vi "LJStreamM.vi"() -> ()   [LabVIEW 2025]
uses:
  LJstreamM globals.vi
panel:
  out "Meter 8":dbl(knob) scale=0.0..1000.0
  out "Meter 7":dbl(knob) scale=0.0..1000.0
  out "Meter 6":dbl(knob) scale=0.0..1000.0
  out "Meter 5":dbl(knob) scale=0.0..1000.0
  out "Meter 4":dbl(knob) scale=0.0..1000.0
  out "Meter 3":dbl(knob) scale=0.0..1000.0
  out "Meter 2":dbl(knob) scale=0.0..1000.0
  out "Meter":dbl(knob) scale=0.0..1000.0
  in  "Fire Button":bool
  in  "Open\nSolenoid":bool
  in  "Close Solenoid":bool
  in  "HIGH":dbl=1.0
  in  "Low":dbl
  in  "FIO6":string="FIO6"
  in  "Close\n Button":bool
  in  "PWM Output 1":string="DIO0_EF_CONFIG_A"
  in  "PWM Output 2":string="DIO2_EF_CONFIG_A"
  in  "Close":dbl=125000.0
  in  "Open":dbl=200000.0
  in  "Open Button":bool
  in  "Config Names":string[](array[string])=["AIN0_RANGE", "AIN0_RESOLUTION_INDEX", "DIO0_EF_ENABLE", "DIO_EF_CLOCK0_ENABLE", "DIO_EF_CLOCK0_ROLL_VALUE", "DIO0_EF_INDEX", "DIO_EF_CLOCK0_ENABLE", "DIO0_EF_ENABLE", "DIO2_EF_ENABLE", "DIO2_EF_INDEX", "DIO2_EF_ENABLE"]
  in  "Config Values":dbl[](array[numeric])=[10.0, 0.0, 0.0, 0.0, 800000.0, 0.0, 1.0, 1.0, 0.0, 0.0, 1.0] format="%.2f"
  out "SerialNumber":i32=470023915
  out "ConnType":i32=1
  out "DevType":i32=7
  in  "Select New Configs":bool
  in  "Save Configuration":bool
  out "Last Command-Response Error Message":string="No Error"
  in  "Change Working Directory":bool
  in  "Max File Size (Bytes)":i32=1048576 min=1 max=2000000000
  in  "Graph?":bool[](array[boolean])=[TRUE, TRUE, TRUE, TRUE, TRUE, TRUE, TRUE, TRUE, FALSE, FALSE, FALSE, FALSE, FALSE, FALSE, FALSE, FALSE]
  out "Scaled":dbl[](array[numeric])=[-2747.1556396198275, -2757.890681247711, -2748.909975194931, -2750.96038772583, -2759.144604291916, -2761.5666391944883, -2777.2834499549863, -2778.0301016235353, -10.5811185836792, -10.5811185836792, -10.581039428710938, -10.581039428710938, -10.581039428710938, -10.5811185836792] format="%.6f"
  in  "Scaling Equation":string[](array[string])=["y = 247.67*a - 126.53", "y = 248.78*b - 125.52", "y = 247.97*c- 125.11", "y = 248.16*d - 125.15", "y = 248.89*e - 125.61", "y = 249.1*f - 125.81", "y = 250.54*g - 126.29", "y = 250.62*h - 126.21", "y=i", "y=j", "y=k", "y=l", "y=m", "y=n", "y=o", "y=p"]
  out "Voltage":dbl[](array[numeric])=[-10.5811185836792, -10.5811185836792, -10.5811185836792, -10.5811185836792, -10.5811185836792, -10.5811185836792, -10.5811185836792, -10.581039428710938, -10.5811185836792, -10.5811185836792, -10.581039428710938, -10.581039428710938, -10.581039428710938, -10.5811185836792] format="%.6f"
  in  "Name":string[](array[string])=["AIN0", "AIN1", "AIN2", "AIN3", "AIN4", "AIN5", "AIN6", "AIN7", "AIN8", "AIN9", "AIN10", "AIN11", "AIN12", "AIN13", "AIN14", "AIN15"]
  in  "Disable Scaling*":bool
  in  "exit":bool
  in  "# Scans On Graph":i32=1000 min=0
  in  "# Channels":i32=14 min=1
  out "Waveform Graph":cluster{dbl, dbl, dbl[][]}(graph)
  out "LJMScanBacklog":dbl format="%.2f"
  out "ms Per Loop":u32=479
  out "DeviceScanBacklog":dbl format="%.2f"
  out "# Scans Read":i32=25
  out "# of iterations":i32=1550
  in  "Scan Rate (Hz)":dbl=50.0 format="%.3f"
  out "Current Data File":path=path "none"
  in  "Data File Prefix":string="data"
  in  "Write To File":bool
  in  "start stream":bool caption="Start Stream"
  out "Last Stream Error Message":string="No Error"
  out "App Name":string="LJStreamM"
  out "Device Config File Name":string="LJStreamM.cfg"
  in  "stop stream":bool
  out "Channel Config":T1={"# Channels"=14, "+Ch"=["AIN0", "AIN1", "AIN2", "AIN3", "AIN4", "AIN5", "AIN6", "AIN7", "AIN8", "AIN9", "AIN10", "AIN11", "AIN12", "AIN13", "AIN14", "AIN15"], "-Ch (U3)"=[], "Ranges (UE9)"=[], "Scaling Equation"=["y = 247.67*a - 126.53", "y = 248.78*b - 125.52", "y = 247.97*c- 125.11", "y = 248.16*d - 125.15", "y = 248.89*e - 125.61", "y = 249.1*f - 125.81", "y = 250.54*g - 126.29", "y = 250.62*h - 126.21", "y=i", "y=j", "y=k", "y=l", "y=m", "y=n", "y=o", "y=p"]} {"Ranges (UE9)" items=["LJ_rgBIP5V", "LJ_rgUNI5V", "LJ_rgUNI2P5V", "LJ_rgUNI1P25V", "LJ_rgUNIP625V"]}
  # "To configure inputs,\nexit this program and\nuse Kipling.  To control\nopening, edit the file\nLJStreamM_open.cfg."
  # "*Scaling is computing intensive. If the LJM Backlog is growing, disable scaling."
  # "# Of Iterations"
  # "0"
  # "1"
  # "2"
  # "3"
  # "4"
  # "5"
  # "6"
  # "7"
  # "8"
  # "9"
  # "10"
  # "11"
  # "12"
  # "13"
  # "14"
  # "15"
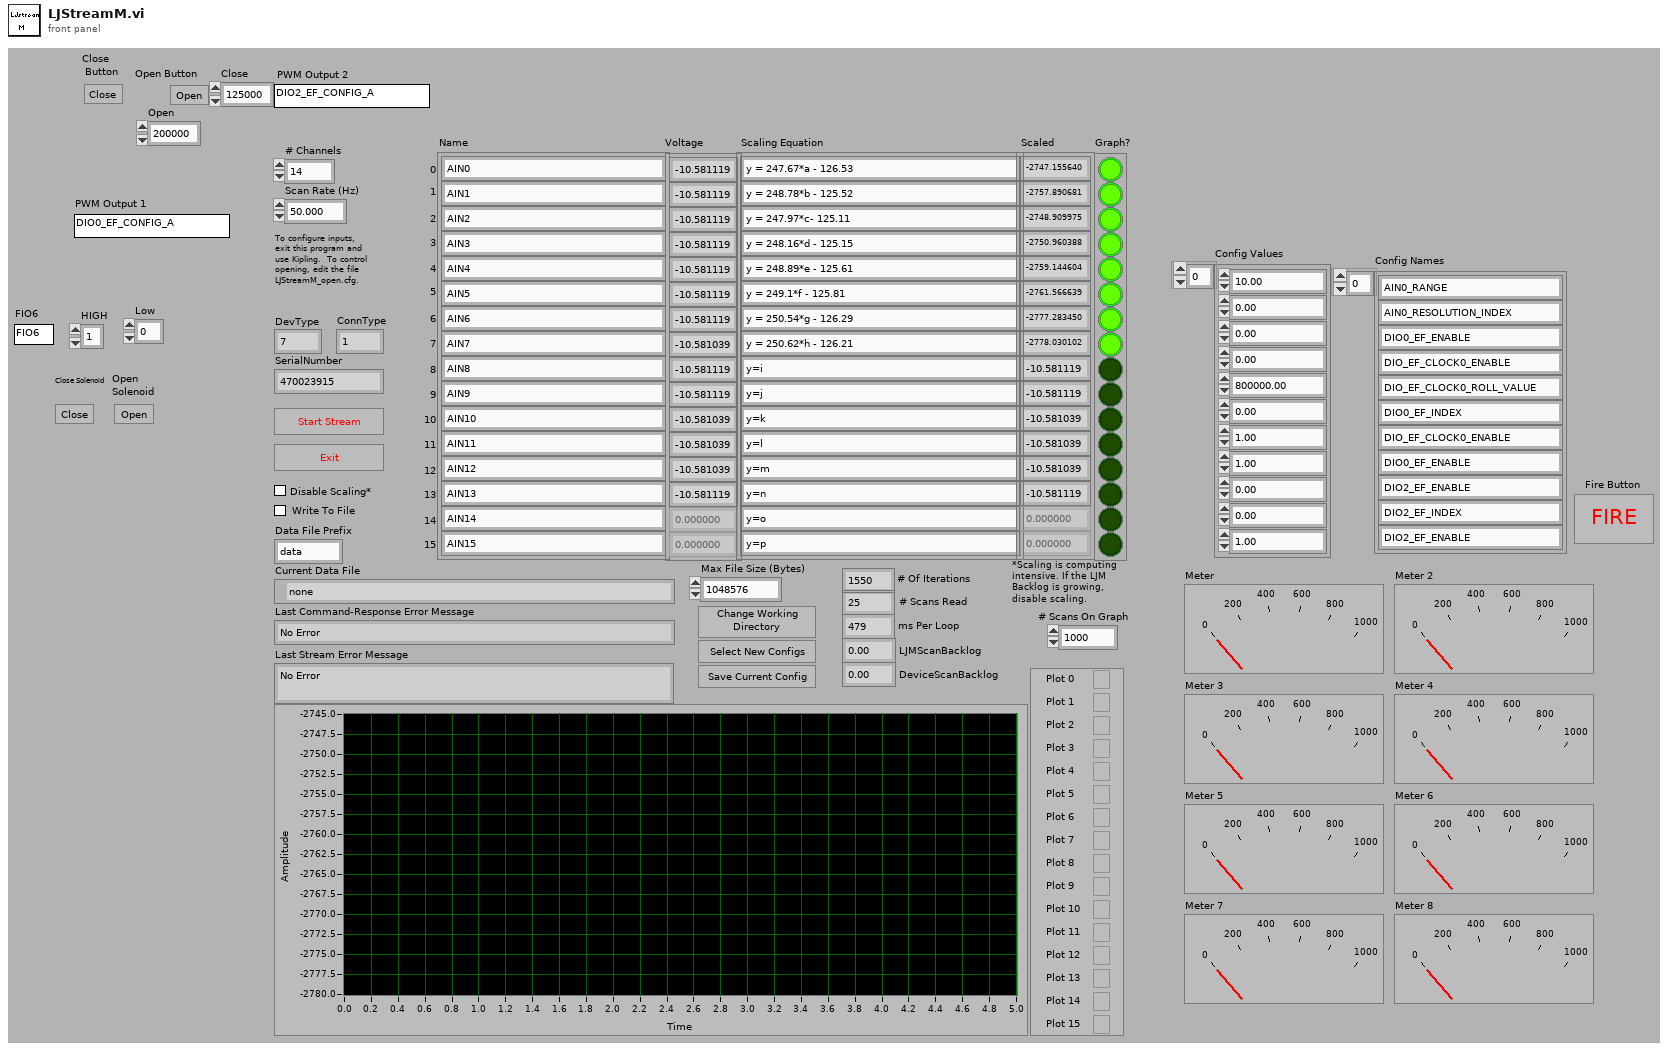
[diagram p1: front panel]
types:
  T1 = cluster{"# Channels":i32, "+Ch":string[], "-Ch (U3)":string[], "Ranges (UE9)":u16[], "Scaling Equation":string[]}
  T2 = cluster{"+Ch":string[], "-Ch":string[], "Ranges":u16[], "Scaling Equation":string[], "Graph?":bool[]}
  T3 = cluster{"DeviceType":string, "ConnectionType":string, "Identifier":string}
  T4 = cluster{"Data File Prefix":string, "Scan Rate (Hz)":dbl, "Graph History":i32, "# Channels":i32, "Disable Scaling":bool, "Max File Size (Bytes)":i32, "Channel Setup":cluster{"+Ch":string[], "-Ch":string[], "Ranges":u16[], "Scaling Equation":string[], "Graph?":bool[]}, "Device Config File Name":string, "Interval (ms)":u32, "Write To File":bool}
  T5 = cluster{"# Channels":i32, "Name":string[], string[], u16[], "Scaling Equation":string[]}
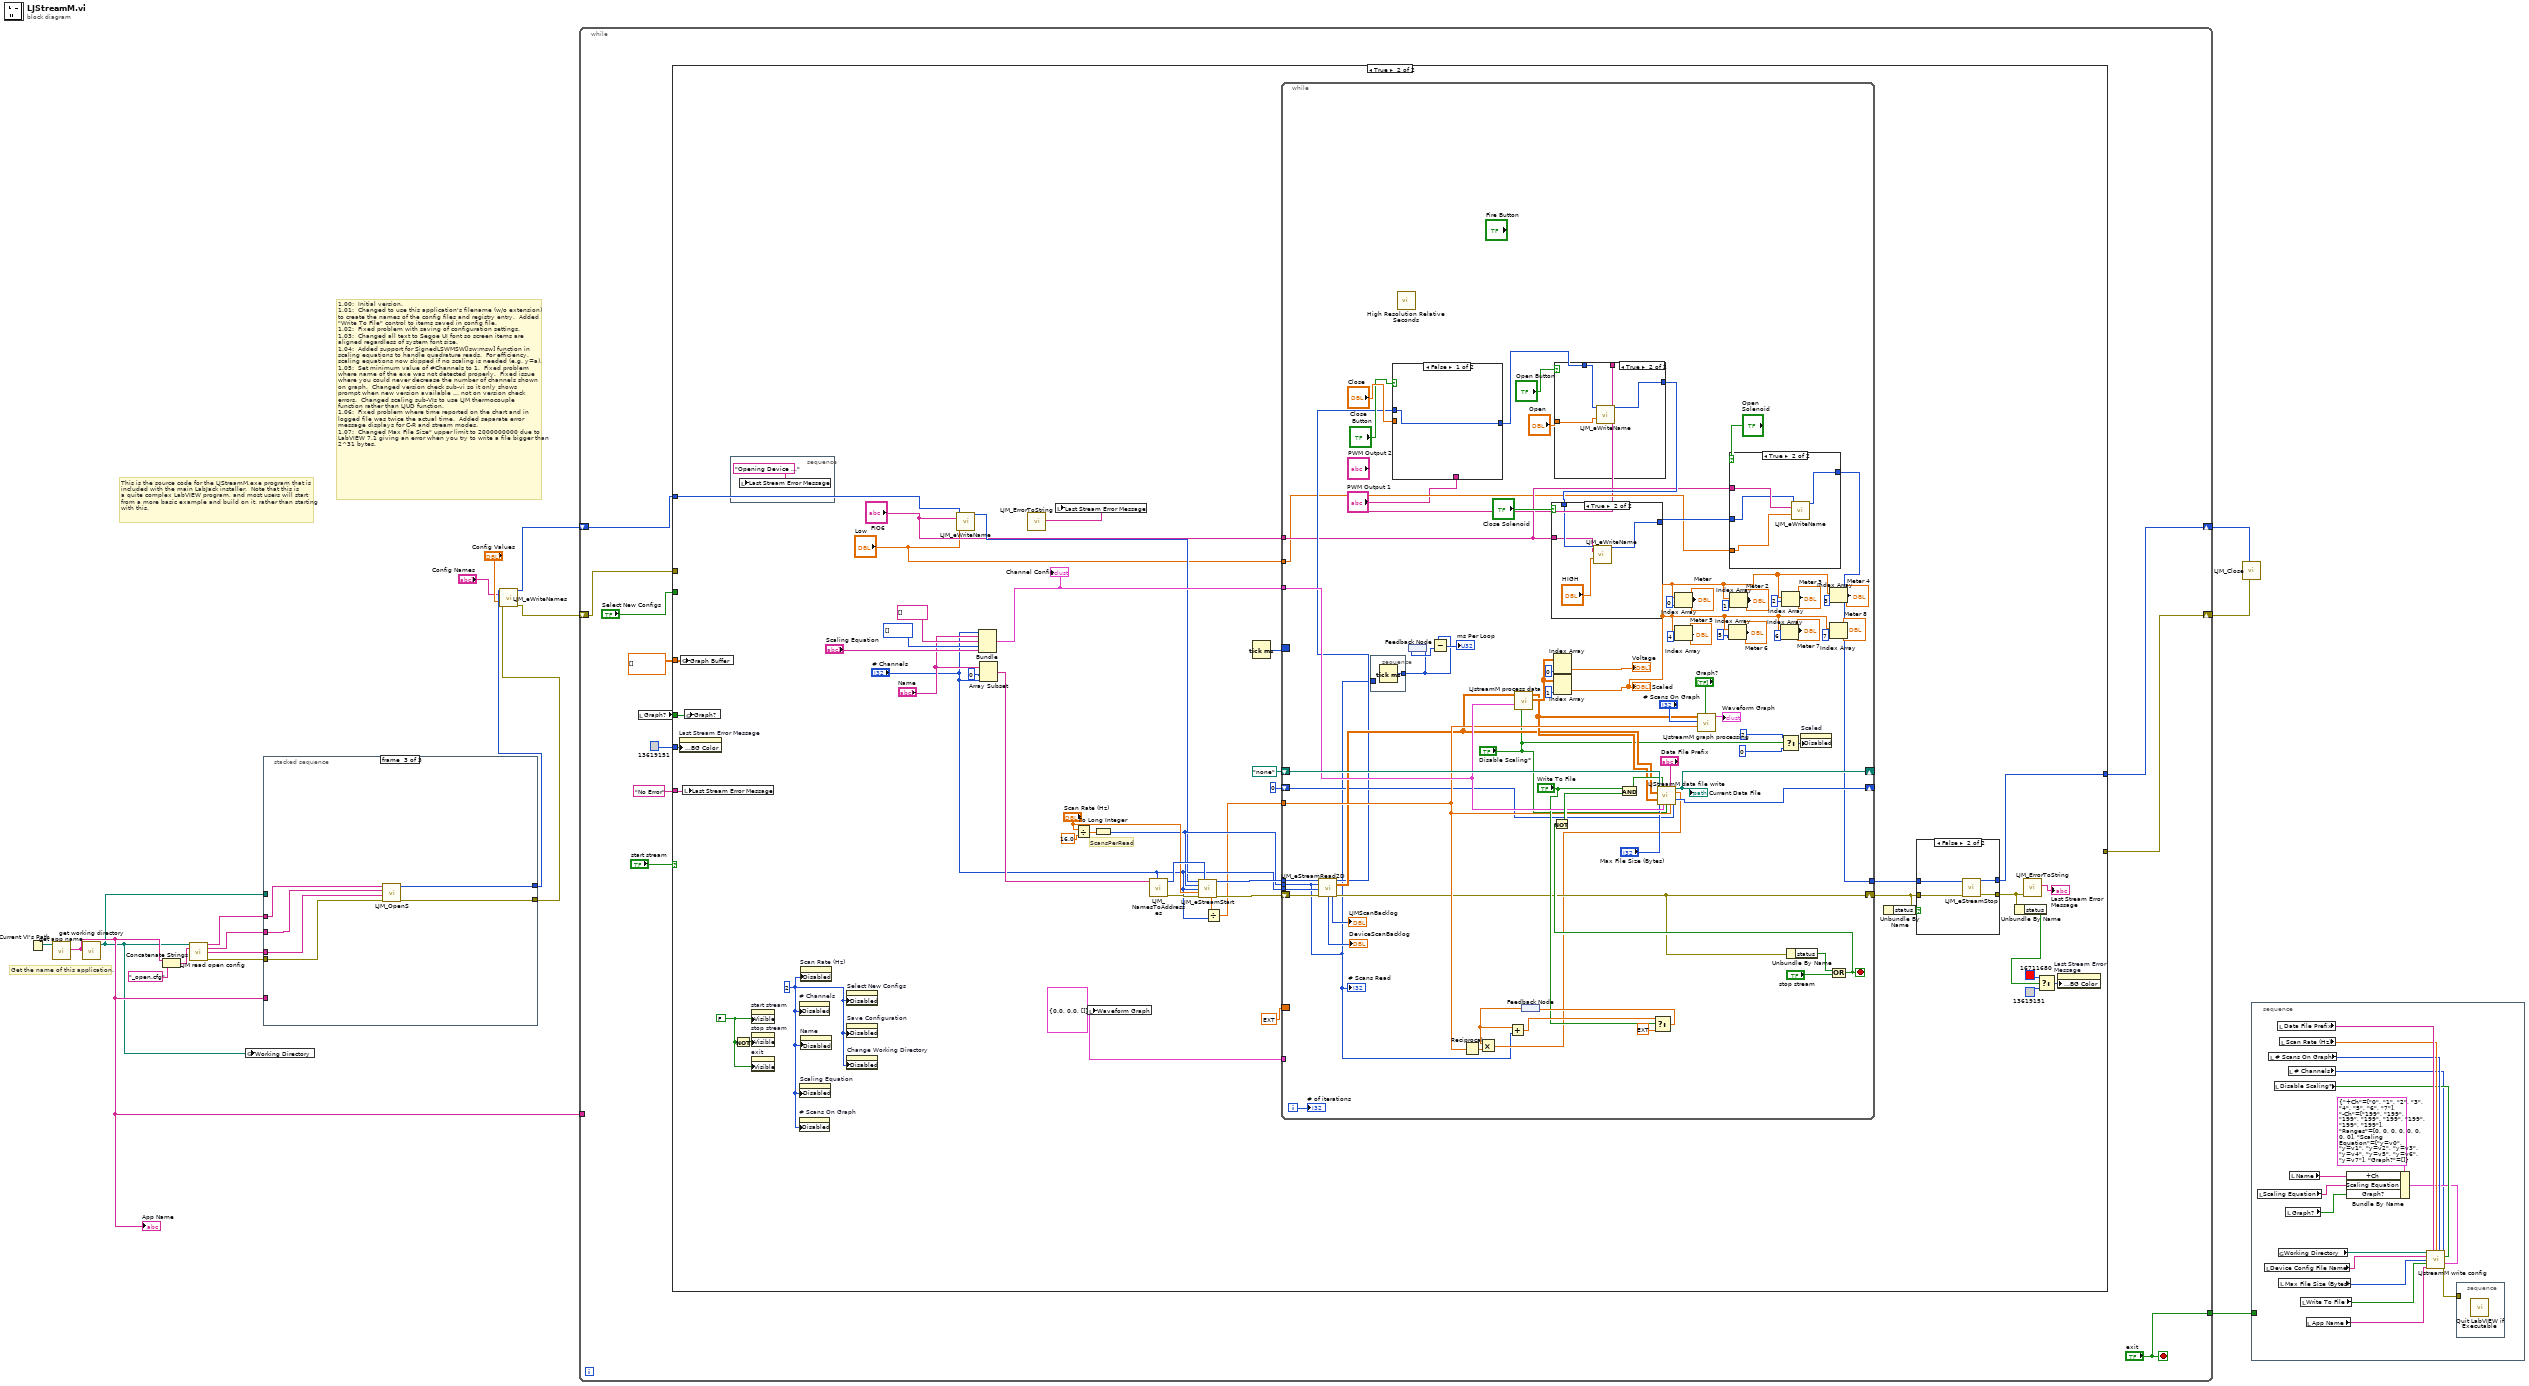
[diagram p0: block diagram]
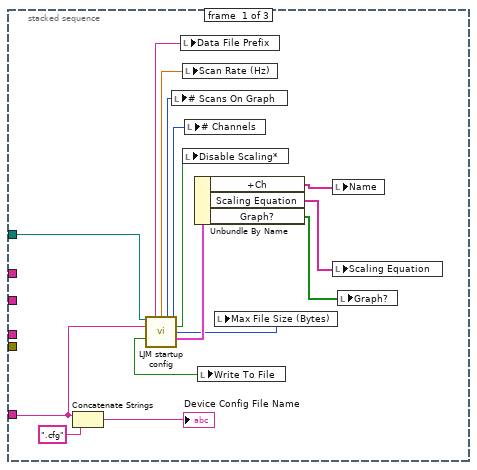
[diagram p2: hidden frame]
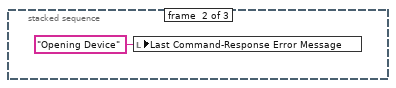
[diagram p3: hidden frame]
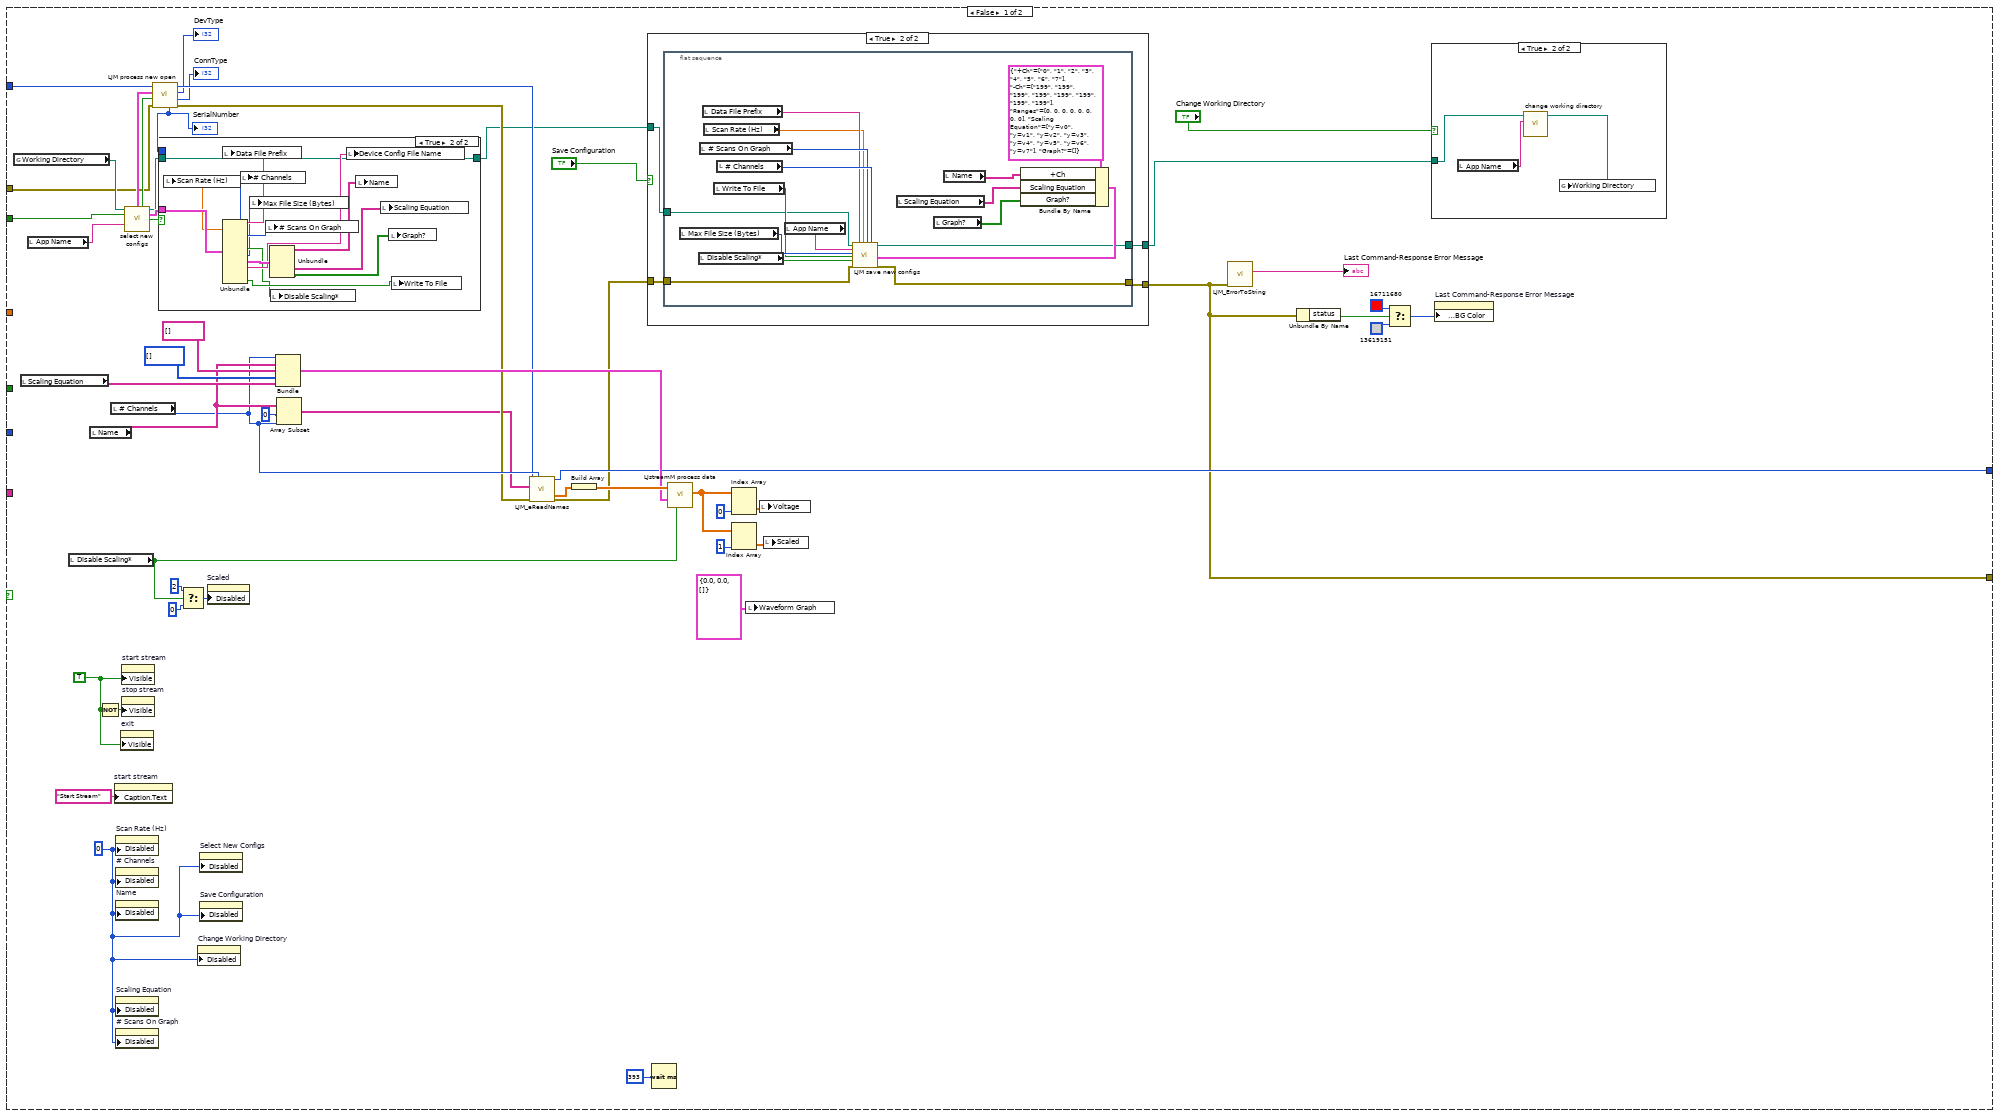
[diagram p4: hidden frame]
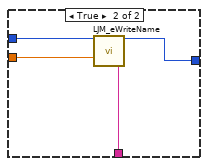
[diagram p10: hidden frame]
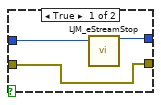
[diagram p12: hidden frame]
diagram:
  # "This is the source code for the LJStreamM.exe program that is\nincluded with the main LabJack installer.  Note that this is \na quite complex LabVIEW program, and most users will start\nfrom a more basic example and build on it, rather than starting\nwith this."
  # "Get the name of this application."
  # "1.00:  Initial version.\n1.01:  Changed to use this application's filename (w/o extension)\nto create the names of the config files and registry entry.  Added\n\"Write To File\" control to items saved in config file.\n1.02:  Fixed problem with saving of configuration settings.\n1.03:  Changed all text to Segoe UI font so screen items are\naligned regardless of system font size.\n1.04:  Added support for SignedLSWMSW[lsw:msw] function in\nscaling equations to handle quadrature reads.  For efficiency,\nscaling equations now skipped if no scaling is needed (e.g. y=a).\n1.05:  Set minimum value of #Channels to 1.  Fixed problem\nwhere name of the exe was not detected properly.  Fixed issue\nwhere you could never decrease the number of channels shown\non graph.  Changed version check sub-vi so it only shows\nprompt when new version available ... not on version check\nerrors.  Changed scaling sub-VIs to use LJM thermocouple\nfunction rather than LJUD function.\n1.06:  Fixed problem where time reported on the chart and in\nlogged file was twice the actual time.  Added separate error\nmessage displays for C-R and stream modes.\n1.07:  Changed Max File Size\" upper limit to 2000000000 due to\nLabVIEW 7.1 giving an error when you try to write a file bigger than\n2^31 bytes."
  n1 = Current VI's Path() -> (path=w17:path)
  n2 = call "get app name.vi"("Current VI's Path"=w17) -> ("App Name Without Extension"=w14:string)  [unwired: 4 in, 2 out]
  "App Name" <- w14
  n3 = call "get working directory.vi"("Application Name"=w14) -> ("Working Directory"=w13:path)  [unwired: 9 in, 1 out]
  n4 = Concatenate Strings(w14, "_open.cfg" ("string")) -> (w15:string)
  n5 = call "LJM read open config.vi"("Working Directory"=w13, "filename"=w15) -> ("DeviceType"=w11:string, "ConnectionType"=w10:string, "Identifier"=w9:string, "error out"=w8:errorcluster)  [unwired: 9 in, 1 out]
  n6 = global write "LJstreamM globals.vi" "Working Directory"(w13) -> ()
  n7 = stacked-sequence {
    tunnel: w14 -> [w19 _ _]
    tunnel: w13 -> [w20 _ _]
    tunnel: w11 -> [_ _ w38]
    tunnel: w10 -> [_ _ w37]
    tunnel: w9 -> [_ _ w36]
    tunnel: w8 -> [_ _ w35]
    tunnel: [_ _ w40] -> w6
    tunnel: [_ _ w39] -> w2
    frame #0 {
      n8 = Concatenate Strings(w19, ".cfg" ("string")) -> (→"Device Config File Name":string)
      n9 = call "LJM startup config.vi"("Working Directory"=w20, "App Name"=w19) -> ("Data File Prefix"=w29:string, "Scan Rate (Hz)"=w23:dbl, "Graph History"=w28:i32, "# Channels"=w27:i32, "Disable Scaling"=w26:bool, "Max File Size (Bytes)"=w25:i32, "Write To File"=w24:bool, "Channel Setup"=w33:T2)  [unwired: 2 in, 4 out]
      n10 = local write "# Scans On Graph"(w28) -> ()
      n11 = local write "Data File Prefix"(w29) -> ()
      n12 = local write "Scan Rate (Hz)"(w23) -> ()
      n13 = local write "Disable Scaling*"(w26) -> ()
      n14 = local write "# Channels"(w27) -> ()
      n15 = Unbundle By Name(w33) -> ("+Ch"=w32:string[], "Scaling Equation"=w31:string[], "Graph?"=w30:bool[])
      n16 = local write "Write To File"(w24) -> ()
      n17 = local write "Max File Size (Bytes)"(w25) -> ()
      n18 = local write "Name"(w32) -> ()
      n19 = local write "Scaling Equation"(w31) -> ()
      n20 = local write "Graph?"(w30) -> ()
    }
    frame #1 {
      n21 = local write "Last Command-Response Error Message"("Opening Device" ("Last Command-Response Error Message")) -> ()
    }
    frame #2 {
      n22 = call <vilib>:"LJM_OpenS.vi"("error in"=w35, "Identifier"=w36, "ConnectionType"=w37, "DeviceType"=w38) -> ("error out"=w39:errorcluster, "Handle"=w40:i32)  [unwired: 6 in]
    }
  }
  n23 = call <vilib>:"LJM_eWriteNames.vi"("Handle In"=w6, "aNames"="Config Names", "aValuesIn"="Config Values", "error in"=w2) -> ("Handle Out"=w5:i32, "error out"=w1:errorcluster)  [unwired: 9 in, 1 out]
  n24 = while {
    tunnel: w14 -> [_]
    tunnel: ["exit"] -> w18
    shift-right: [w45] -> w12
    shift-left: w5 -> [w41]
    shift-right: [w42] -> w7
    shift-left: w1 -> [w44]
    stop <- "exit" stop-if-true
    n25 = local read "Graph?"() -> (w48:bool[])
    n26 = case shown="True" "start stream" {
      tunnel: dbl[][] [] ("Graph Buffer") -> [_ w180]
      tunnel: w48 -> [_ w179]
      tunnel: u32 13619151 -> [_ w173]
      tunnel: [w58 _] -> w42
      tunnel: [w87 w158] -> w45
      tunnel: "No Error" ("Last Stream Error Message") -> [_ w154]
      tunnel: w41 -> [w80 w149]
      tunnel: w44 -> [w53 _]
      tunnel: "Select New Configs" -> [w52 _]
      frame False {
        w84 = TRUE ("Visible")
        w64 = u8 0 ("Disabled")
        n27 = global read "LJstreamM globals.vi" "Working Directory"() -> (w66:path)
        n28 = local read "Scaling Equation"() -> (w91:string[])
        n29 = local read "App Name"() -> (w81:string)
        n30 = local read "Disable Scaling*"() -> (w68:bool)
        n31 = local read "Name"() -> (w90:string[])
        n32 = Not(x=w84) -> (.not. x?=w102:bool)
        n33 = local read "# Channels"() -> (w82:i32)
        n34 = property on="start stream" class="Bool"("Caption.Text"="Start Stream") -> ()  [unwired: 2 in, 2 out]
        n35 = property on="Scan Rate (Hz)" class="DigNum (strict)"("Disabled"=w64) -> ()  [unwired: 2 in, 2 out]
        n36 = property on="# Channels" class="DigNum (strict)"("Disabled"=w64) -> ()  [unwired: 2 in, 2 out]
        n37 = property on="Name" class="Arr (strict)"("Disabled"=w64) -> ()  [unwired: 2 in, 2 out]
        n38 = property on="Scaling Equation" class="Arr (strict)"("Disabled"=w64) -> ()  [unwired: 2 in, 2 out]
        n39 = property on="# Scans On Graph" class="DigNum (strict)"("Disabled"=w64) -> ()  [unwired: 2 in, 2 out]
        n40 = property on="exit" class="Bool"("Visible"=w84) -> ()  [unwired: 2 in, 2 out]
        n41 = property on="start stream" class="Bool"("Visible"=w84) -> ()  [unwired: 2 in, 2 out]
        n42 = property on="stop stream" class="Bool"("Visible"=w102) -> ()  [unwired: 2 in, 2 out]
        n43 = call "select new configs.vi"("Current Working Dir"=w66, "Select New Configs"=w52, "App Name"=w81) -> ("Open Configs"=w78:T3, "New Open Config?"=w79:bool, "Working Dir Out"=w73:path, "Exp Configs"=w74:T4, "New Exp Config?"=w75:bool)  [unwired: 8 in]
        n44 = call "LJM process new open.vi"("error in"=w53, "Open New Device?"=w79, "Open Configs"=w78, "Handle"=w80) -> ("error out"=w76:errorcluster, "ConnType"=→"ConnType":i32, "DevType"=→"DevType":i32, "Handle Out"=w77:i32, "SerialNumber"=w54:i32)  [unwired: 3 in]
        "SerialNumber" <- w54
        n45 = case shown="True" w75 {
          tunnel: w74 -> [_ w111]
          tunnel: w73 -> [w104 w108]
          tunnel: [w104 w108] -> w72
          tunnel: w54 -> [_ _]
          frame False {
          }
          frame True {
            n46 = Unbundle(w111) -> ("Data File Prefix"=w118:string, "Scan Rate (Hz)"=w109:dbl, "Graph History"=w106:i32, "# Channels"=w107:i32, "Disable Scaling"=w110:bool, "Max File Size (Bytes)"=w105:i32, "Channel Setup"=w116:T2, "Device Config File Name"=w112:string, "Write To File"=w117:bool)  [unwired: 1 out]
            n47 = local write "Scan Rate (Hz)"(w109) -> ()
            n48 = local write "Data File Prefix"(w118) -> ()
            n49 = local write "# Channels"(w107) -> ()
            n50 = local write "Max File Size (Bytes)"(w105) -> ()
            n51 = local write "# Scans On Graph"(w106) -> ()
            n52 = Unbundle(w116) -> ("+Ch"=w113:string[], "Scaling Equation"=w114:string[], "Graph?"=w115:bool[])  [unwired: 2 out]
            n53 = local write "Disable Scaling*"(w110) -> ()
            n54 = local write "Device Config File Name"(w112) -> ()
            n55 = local write "Name"(w113) -> ()
            n56 = local write "Scaling Equation"(w114) -> ()
            n57 = local write "Graph?"(w115) -> ()
            n58 = local write "Write To File"(w117) -> ()
          }
        }
        n59 = Select(t=u8 2, s=w68, f=u8 0) -> (s? t:f=w71:u8)
        n60 = property on="Change Working Directory" class="Bool"("Disabled"=w64) -> ()  [unwired: 2 in, 2 out]
        n61 = property on="Select New Configs" class="Bool"("Disabled"=w64) -> ()  [unwired: 2 in, 2 out]
        n62 = property on="Save Configuration" class="Bool"("Disabled"=w64) -> ()  [unwired: 2 in, 2 out]
        n63 = property on="Scaled" class="Arr (strict)"("Disabled"=w71) -> ()  [unwired: 2 in, 2 out]
        n64 = Bundle("# Channels"=w82, "Name"=w90, string[] [], u16[] [], "Scaling Equation"=w91) -> (w88:T5)  [unwired: 1 in]
        n65 = Array Subset(array=w90, index=0 ("Array Index"), length=w82) -> (w67:string[])
        n66 = call <vilib>:"LJM_eReadNames.vi"("Handle In"=w77, "NumFrames (Auto-Detect)"=w82, "aNames"=w67, "error in"=w76) -> ("Handle Out"=w87:i32, "aValuesOut"=w95:dbl[], "error out"=w83:errorcluster)  [unwired: 8 in, 1 out]
        n67 = Build Array(w95) -> (w89:dbl[][])
        n68 = case shown="True" "Save Configuration" {
          tunnel: w83 -> [w120 w124]
          tunnel: [w120 w123] -> w58
          tunnel: w72 -> [w119 w122]
          tunnel: [w119 w121] -> w65
          frame False {
          }
          frame True {
            n69 = flat-sequence {
              tunnel: w124 -> [w131]
              tunnel: [w134] -> w123
              tunnel: w122 -> [w126]
              tunnel: [w125] -> w121
              frame #0 {
                n70 = local read "Max File Size (Bytes)"() -> (w130:i32)
                n71 = local read "Disable Scaling*"() -> (w129:bool)
                n72 = local read "# Scans On Graph"() -> (w136:i32)
                n73 = local read "Data File Prefix"() -> (w135:string)
                n74 = local read "Scan Rate (Hz)"() -> (w132:dbl)
                n75 = local read "Write To File"() -> (w128:bool)
                n76 = local read "# Channels"() -> (w137:i32)
                n77 = local read "App Name"() -> (w127:string)
                n78 = local read "Scaling Equation"() -> (w140:string[])
                n79 = local read "Graph?"() -> (w141:bool[])
                n80 = local read "Name"() -> (w139:string[])
                n81 = Bundle By Name(cluster=T2 {"+Ch"=["0", "1", "2", "3", "4", "5", "6", "7"], "-Ch"=["199", "199", "199", "199", "199", "199", "199", "199"], "Ranges"=[0, 0, 0, 0, 0, 0, 0, 0], "Scaling Equation"=["y=v0", "y=v1", "y=v2", "y=v3", "y=v4", "y=v5", "y=v6", "y=v7"], "Graph?"=[]} ("Channel Setup"), "+Ch"=w139, "Scaling Equation"=w140, "Graph?"=w141) -> (w133:T2)
                n82 = call "LJM save new configs.vi"("Working Directory"=w126, "App name"=w127, "Max File Size (Bytes)"=w130, "Write To File"=w128, "Disable Scaling"=w129, "error in"=w131, "Data File Prefix"=w135, "Scan Rate (Hz)"=w132, "Graph History"=w136, "# Channels"=w137, "Channel Setup"=w133) -> ("Working Directory Out"=w125:path, "error out"=w134:errorcluster)  [unwired: 7 in]
              }
            }
          }
        }
        n83 = Wait (ms)(milliseconds to wait=u32 393) -> ()  [unwired: 1 out]
        n84 = call "LJstreamM process data.vi"("Disable Scaling"=w68, "Channel Config"=w88, "Voltages"=w89) -> ("Volts,Scaled Averages"=w99:dbl[][])  [unwired: 7 in, 1 out]
        n85 = Index Array(array=w99, index (col)=0 ("Disabled Index (col)")) -> (element=w98:dbl[])  [unwired: 1 in]
        n86 = Index Array(array=w99, index (col)=1 ("Disabled Index (col)")) -> (element=w97:dbl[])  [unwired: 1 in]
        n87 = local write "Waveform Graph"(cluster{dbl, dbl, dbl[][]} {0.0, 0.0, []} ("Waveform Graph")) -> ()
        n88 = local write "Voltage"(w98) -> ()
        n89 = local write "Scaled"(w97) -> ()
        n90 = call <vilib>:"LJM_ErrorToString.vi"("error in"=w58) -> ("String"=→"Last Command-Response Error Message":string)  [unwired: 10 in]
        n91 = Unbundle By Name(w58) -> ("status"=w57:bool)
        n92 = Select(t=u32 16711680, s=w57, f=u32 13619151) -> (s? t:f=w59:u32)
        n93 = case shown="True" "Change Working Directory" {
          tunnel: w65 -> [_ w142]
          frame False {
          }
          frame True {
            n94 = local read "App Name"() -> (w143:string)
            n95 = call "change working directory.vi"("Application Name"=w143, "Working Directory In"=w142) -> ("Working Directory Out"=w144:path)  [unwired: 9 in]
            n96 = global write "LJstreamM globals.vi" "Working Directory"(w144) -> ()
          }
        }
        n97 = property on="Last Command-Response Error Message" class="Str"("Text.Text Colors:BG Color"=w59) -> ()  [unwired: 2 in, 2 out]
      }
      frame True {
        w151 = FALSE ("Visible")
        w150 = u8 2 ("Disabled")
        w182 = cluster{dbl, dbl, dbl[][]} {0.0, 0.0, []} ("Waveform Graph")
        # "ScansPerRead"
        n98 = property on="Last Stream Error Message" class="Str"("Text.Text Colors:BG Color"=w173) -> ()  [unwired: 2 in, 2 out]
        n99 = global write "LJstreamM globals.vi" "Graph Buffer"(w180) -> ()
        n100 = local write "Last Stream Error Message"(w154) -> ()
        n101 = global write "LJstreamM globals.vi" "Graph?"(w179) -> ()
        n102 = stacked-sequence {
          frame #0 {
            n103 = local write "Last Stream Error Message"("Opening Device ..." ("Error Message")) -> ()
          }
        }
        n104 = Not(x=w151) -> (.not. x?=w181:bool)
        n105 = property on="start stream" class="Bool"("Visible"=w151) -> ()  [unwired: 2 in, 2 out]
        n106 = property on="stop stream" class="Bool"("Visible"=w181) -> ()  [unwired: 2 in, 2 out]
        n107 = property on="exit" class="Bool"("Visible"=w151) -> ()  [unwired: 2 in, 2 out]
        n108 = property on="# Channels" class="DigNum (strict)"("Disabled"=w150) -> ()  [unwired: 2 in, 2 out]
        n109 = property on="# Scans On Graph" class="DigNum (strict)"("Disabled"=w150) -> ()  [unwired: 2 in, 2 out]
        n110 = property on="Scaling Equation" class="Arr (strict)"("Disabled"=w150) -> ()  [unwired: 2 in, 2 out]
        n111 = property on="Scan Rate (Hz)" class="DigNum (strict)"("Disabled"=w150) -> ()  [unwired: 2 in, 2 out]
        n112 = property on="Name" class="Arr (strict)"("Disabled"=w150) -> ()  [unwired: 2 in, 2 out]
        n113 = property on="Select New Configs" class="Bool"("Disabled"=w150) -> ()  [unwired: 2 in, 2 out]
        n114 = property on="Save Configuration" class="Bool"("Disabled"=w150) -> ()  [unwired: 2 in, 2 out]
        n115 = property on="Change Working Directory" class="Bool"("Disabled"=w150) -> ()  [unwired: 2 in, 2 out]
        n116 = call <vilib>:"LJM_eWriteName.vi"("Handle In"=w149, "Name"="FIO6", "Value"="Low") -> ("Handle Out"=w148:i32)  [unwired: 11 in, 1 out]
        n117 = Bundle("# Channels"="# Channels", "Name"="Name", string[] [], u16[] [], "Scaling Equation"="Scaling Equation") -> (w167:T5)  [unwired: 1 in]
        "Channel Config" <- w167
        n118 = Array Subset(array="Name", index=0 ("Array Index"), length="# Channels") -> (w165:string[])
        n119 = call <vilib>:"LJM_ErrorToString.vi"() -> ("String"=w153:string)  [unwired: 11 in]
        n120 = local write "Last Stream Error Message"(w153) -> ()
        n121 = Divide(x="Scan Rate (Hz)", y=16.0) -> (x/y=w161:dbl)
        n122 = local write "Waveform Graph"(w182) -> ()
        n123 = To Long Integer(number=w161) -> (32bit integer=w160:i32)
        n124 = call <vilib>:"LJM_NamesToAddresses.vi"("NumFrames (Auto-Detect)"="# Channels", "aNames"=w165) -> ("error out"=w166:errorcluster, "aAddresses"=w164:i32[])  [unwired: 7 in, 1 out]
        n125 = call <vilib>:"LJM_eStreamStart.vi"("Handle In"=w148, "aScanList"=w164, "ScansPerRead"=w160, "NumAddresses (-1 = Auto-Detect)"="# Channels", "ScanRate"="Scan Rate (Hz)", "error in"=w166) -> ("Handle Out"=w187:i32, "Actual SampleRate"=w157:dbl, "error out"=w185:errorcluster)  [unwired: 4 in, 3 out]
        n126 = Divide(x=w157, y="# Channels") -> (x/y=w155:dbl)
        n127 = Tick Count (ms)() -> (millisecond timer value=w145:u32)
        n128 = while {
          shift-left: u32 0 ("Data File #") -> [w220]
          shift-right: [w232] -> _
          tunnel: w182 -> [_]
          tunnel: w167 -> [w250]
          shift-left: w185 -> [w259]
          shift-right: [w230] -> w184
          tunnel: [w215] -> w188
          tunnel: w155 -> [w243]
          shift-left: path "none" ("Current Data File Out") -> [w257]
          shift-right: [w258] -> _
          tunnel: w187 -> [w263]
          tunnel: w160 -> [w192]
          tunnel: "# Channels" -> [w229]
          border: ext 0.0 -> [_]
          border: w145 -> [_]
          tunnel: "FIO6" -> [w214]
          tunnel: "Low" -> [w213]
          i -> [w262]
          stop <- w240 stop-if-true
          n129 = call <vilib>:"LJM_eStreamRead2D.vi"("Handle In"=w263, "ScansPerRead"=w192, "NumAddresses"=w229, "error in"=w259) -> ("Handle Out"=w219:i32, "aData Out"=w231:dbl[][], "DeviceScanBacklog"=→"DeviceScanBacklog":i32, "LJMScanBacklog"=→"LJMScanBacklog":i32, "error out"=w230:errorcluster)  [unwired: 7 in]
          n130 = stacked-sequence {
            tunnel: w192 -> [_]
            tunnel: [w286] -> w193
            frame #0 {
              n131 = Tick Count (ms)() -> (millisecond timer value=w286:u32)
            }
          }
          n132 = case shown="False" "Close\n Button" {
            tunnel: "Close" -> [_ w280]
            tunnel: "PWM Output 1" -> [_ w279]
            tunnel: w219 -> [w276 w278]
            tunnel: [w276 w277] -> w223
            frame False {
            }
            frame True {
              n133 = call <vilib>:"LJM_eWriteName.vi"("Handle In"=w278, "Name"=w279, "Value"=w280) -> ("Handle Out"=w277:i32)  [unwired: 11 in, 1 out]
            }
          }
          n134 = call <vilib>:"High Resolution Relative Seconds.vi"() -> ()  [unwired: 1 out]
          n135 = feedback-in #1(w193) -> ()
          n136 = feedback #1() -> (w261:u32)
          n137 = Subtract(x=w193, y=w261) -> (x-y=→"ms Per Loop":u32)
          n138 = Reciprocal(x=w243) -> (1/x=w249:dbl)
          n139 = call "LJstreamM process data.vi"("Disable Scaling"="Disable Scaling*", "Channel Config"=w250, "Voltages"=w231) -> ("Volts,Scaled Averages"=w239:dbl[][], "Scaled Data"=w238:dbl[][])  [unwired: 7 in]
          n140 = feedback #2() -> (w245:ext)
          n141 = Multiply(x=w245, y=w249) -> (x*y=w194:ext)
          n142 = Add(x=w245, y=w192) -> (x+y=w247:ext)
          n143 = Index Array(array=w239, index (col)=0 ("Disabled Index (col)")) -> (element=→"Voltage":dbl[])  [unwired: 1 in]
          n144 = Index Array(array=w239, index (col)=1 ("Disabled Index (col)")) -> (element=w195:dbl[])  [unwired: 1 in]
          "Scaled" <- w195
          n145 = case shown="True" "Open Button" {
            tunnel: "Open" -> [_ w285]
            tunnel: "PWM Output 1" -> [_ w284]
            tunnel: w223 -> [w281 w283]
            tunnel: [w281 w282] -> w218
            frame False {
            }
            frame True {
              n146 = call <vilib>:"LJM_eWriteName.vi"("Handle In"=w283, "Name"=w284, "Value"=w285) -> ("Handle Out"=w282:i32)  [unwired: 11 in, 1 out]
            }
          }
          n147 = case shown="True" "Close Solenoid" {
            tunnel: w218 -> [w271 w274]
            tunnel: [w271 w275] -> w216
            tunnel: w214 -> [_ w273]
            frame False {
            }
            frame True {
              n148 = call <vilib>:"LJM_eWriteName.vi"("Handle In"=w274, "Name"=w273, "Value"="HIGH") -> ("Handle Out"=w275:i32)  [unwired: 11 in, 1 out]
            }
          }
          n149 = Select(t=w247, s="Write To File", f=ext 0.0) -> (s? t:f=w246:ext)
          n150 = feedback-in #2(w246) -> ()
          n151 = Index Array(array=w195, index=u8 0 ("t")) -> (element=→"Meter":dbl)
          n152 = Index Array(array=w195, index=u8 4 ("t")) -> (element=→"Meter 5":dbl)
          n153 = call "LJstreamM graph processing.vi"("Graph?"="Graph?", "Scan Rate"=w243, "Graph History (# scans)"="# Scans On Graph", "Scaled Data"=w238) -> ("Graph Data"=→"Waveform Graph":cluster{dbl, dbl, dbl[][]})  [unwired: 7 in]
          n154 = Index Array(array=w195, index=u8 5 ("t")) -> (element=→"Meter 6":dbl)
          n155 = case shown="True" "Open\nSolenoid" {
            tunnel: [w266 w270] -> w215
            tunnel: w214 -> [_ w269]
            tunnel: w216 -> [w266 w268]
            tunnel: w213 -> [_ w267]
            frame False {
            }
            frame True {
              n156 = call <vilib>:"LJM_eWriteName.vi"("Handle In"=w268, "Name"=w269, "Value"=w267) -> ("Handle Out"=w270:i32)  [unwired: 11 in, 1 out]
            }
          }
          n157 = Index Array(array=w195, index=u8 1 ("t")) -> (element=→"Meter 2":dbl)
          n158 = Index Array(array=w195, index=u8 6 ("t")) -> (element=→"Meter 7":dbl)
          n159 = Index Array(array=w195, index=u8 2 ("t")) -> (element=→"Meter 3":dbl)
          n160 = Select(t=u8 2, s="Disable Scaling*", f=u8 0) -> (s? t:f=w236:u8)
          n161 = Unbundle By Name(w230) -> ("status"=w241:bool)
          n162 = property on="Scaled" class="Arr (strict)"("Disabled"=w236) -> ()  [unwired: 2 in, 2 out]
          n163 = Index Array(array=w195, index=u8 7 ("t")) -> (element=→"Meter 8":dbl)
          n164 = Index Array(array=w195, index=u8 3 ("t")) -> (element=→"Meter 4":dbl)
          n165 = Compound Arithmetic op=OR(w241, "stop stream") -> (w240:bool)
          n166 = Not(x=w240) -> (.not. x?=w264:bool)
          n167 = And(x="Write To File", y=w264) -> (x .and. y?=w256:bool)
          n168 = call "LJStreamM data file write.vi"("Current Data File In"=w257, "Write To File"=w256, "Data File Prefix"="Data File Prefix", "Voltages"=w231, "Time"=w194, "Scaled Data"=w238, "max file size (bytes)"="Max File Size (Bytes)", "Channel Config"=w250, "Disable Scaling"="Disable Scaling*", "Scan Rate"=w243, "Starting #"=w220) -> ("Current Data File Out"=w258:path, "Data File #"=w232:u32)  [unwired: 3 in]
          "Current Data File" <- w258
          "# of iterations" <- w262
          "# Scans Read" <- w192
        }
        n169 = Unbundle By Name(w184) -> ("status"=w186:bool)
        n170 = case shown="False" w186 {
          tunnel: w188 -> [w289 w293]
          tunnel: [w288 w292] -> w159
          tunnel: w184 -> [w288 w291]
          tunnel: [w287 w290] -> w158
          frame True {
            n171 = call <vilib>:"LJM_eStreamStop.vi"("Handle In"=w289) -> ("Handle Out"=w287:i32)  [unwired: 13 in, 1 out]
          }
          frame False {
            n172 = call <vilib>:"LJM_eStreamStop.vi"("Handle In"=w293, "error in"=w291) -> ("Handle Out"=w290:i32, "error out"=w292:errorcluster)  [unwired: 12 in]
          }
        }
        n173 = Unbundle By Name(w159) -> ("status"=w175:bool)
        n174 = call <vilib>:"LJM_ErrorToString.vi"("error in"=w159) -> ("String"=→"Last Stream Error Message":string)  [unwired: 10 in]
        n175 = Select(t=u32 16711680, s=w175, f=u32 13619151) -> (s? t:f=w174:u32)
        n176 = property on="Last Stream Error Message" class="Str"("Text.Text Colors:BG Color"=w174) -> ()  [unwired: 2 in, 2 out]
      }
    }
  }
  n177 = call <vilib>:"LJM_Close.vi"("error in"=w7, "Handle"=w12) -> ()  [unwired: 9 in, 1 out]
  n178 = stacked-sequence {
    tunnel: w18 -> [_]
    frame #0 {
      n179 = local read "Scaling Equation"() -> (w302:string[])
      n180 = local read "Device Config File Name"() -> (w297:string)
      n181 = local read "# Scans On Graph"() -> (w306:i32)
      n182 = local read "Disable Scaling*"() -> (w305:bool)
      n183 = local read "Data File Prefix"() -> (w308:string)
      n184 = global read "LJstreamM globals.vi" "Working Directory"() -> (w296:path)
      n185 = local read "Max File Size (Bytes)"() -> (w299:i32)
      n186 = local read "Scan Rate (Hz)"() -> (w307:dbl)
      n187 = local read "Graph?"() -> (w301:bool[])
      n188 = local read "# Channels"() -> (w294:i32)
      n189 = local read "Name"() -> (w303:string[])
      n190 = local read "Write To File"() -> (w298:bool)
      n191 = local read "App Name"() -> (w295:string)
      n192 = Bundle By Name(cluster=T2 {"+Ch"=["0", "1", "2", "3", "4", "5", "6", "7"], "-Ch"=["199", "199", "199", "199", "199", "199", "199", "199"], "Ranges"=[0, 0, 0, 0, 0, 0, 0, 0], "Scaling Equation"=["y=v0", "y=v1", "y=v2", "y=v3", "y=v4", "y=v5", "y=v6", "y=v7"], "Graph?"=[]} ("Channel Setup"), "+Ch"=w303, "Scaling Equation"=w302, "Graph?"=w301) -> (w300:T2)
      n193 = call "LJstreamM write config.vi"("Working Directory"=w296, "Data File Prefix"=w308, "Scan Rate (Hz)"=w307, "Graph History"=w306, "# Channels"=w294, "filename"=w297, "Disable Scaling"=w305, "Max File Size (Bytes)"=w299, "Write To File"=w298, "Channel Setup"=w300, "App Name"=w295) -> ("error out"=w309:errorcluster)  [unwired: 4 in]
      n194 = stacked-sequence {
        tunnel: w309 -> [_]
        frame #0 {
          n195 = call "Quit LabVIEW if Executable.vi"() -> ()  [unwired: 1 in]
        }
      }
    }
  }
